vi "Set Group Acceleration.vi"(4 "error in (no error)":errorcluster, 5 "Acceleration (0 units/s²)":dbl min=0.0 format="%.6g", 6 "Group Number (1)":i32=1 min=1, 7 "VISA resource name":refnum<visa-resource-name>) -> (0 "error out":errorcluster, 3 "VISA resource name out":refnum<visa-resource-name>)   [LabVIEW 2014, in "Newport ESP301.lvlib"]
doc: "This command is used to set the vectorial acceleration value for a group. This value will be used during coordinated motion of axes assigned to the group. It will override any original acceleration values specified for individual axes using AC command. The axes’ original values will be restored when the group to which they have been assigned is deleted.\nThis command takes effect immediately. It can be executed when controller is idling or motion is in progress or inside a program.\n<B>Note:</B>\nAvoid changing acceleration during acceleration or deceleration phases of a move. For better predictable results, change acceleration only when all the axes assigned to this group are not in motion."
uses:
  Newport ESP301.lvlib
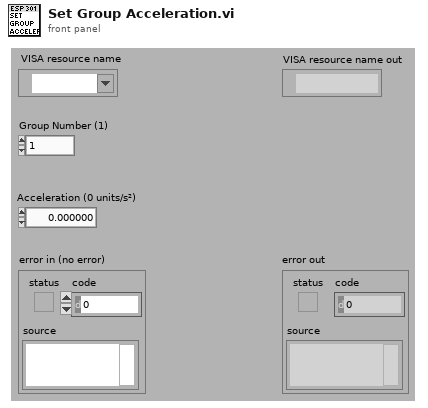
[diagram p1: front panel]
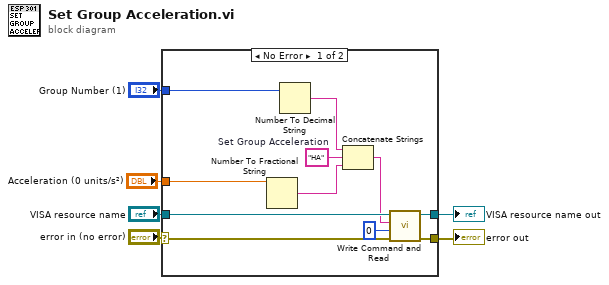
[diagram p0: block diagram]
diagram:
  n1 = case shown="No Error" "error in (no error)" {
    selector: "error in (no error)" -> [w14 w19]
    tunnel: [w16 w19] -> w6
    tunnel: "VISA resource name" -> [w17 w18]
    tunnel: [w15 w18] -> w5
    tunnel: "Group Number (1)" -> [w10 _]
    tunnel: "Acceleration (0 units/s²)" -> [w7 _]
    frame No Error {
      w13 = "HA"  # Set Group Acceleration
      n2 = Number To Fractional String(number=w7) -> (F-format string=w8:string)  [unwired: 1 in, 2 out]
      n3 = Number To Decimal String(number=w10) -> (decimal integer string=w12:string)  [unwired: 1 in]
      n4 = Concatenate Strings(w12, w13, w8) -> (w11:string)
      n5 = call "Write Command and Read.vi"("error in (no error)"=w14, "Bytes to read (100)"=u32 0, "Command"=w11, "VISA resource name"=w17) -> ("error out"=w16:errorcluster, "VISA resource name out"=w15:refnum<visa-resource-name>)  [unwired: 3 in, 1 out]
    }
    frame Error {
    }
  }
  "error out" <- w6
  "VISA resource name out" <- w5
